vi "aft_ANC_Analyze Residual Siganl.vi"(10 "restart averaging":bool, 11 "signal":fxp<+/-,24,4>[](array[numeric]) format="%.22g") -> (2 "residual noise":dbl[](array[numeric]), 3 "power spectrum":cluster{"f0":dbl, "df":dbl, "magnitude":dbl[]})   [LabVIEW 2019]
uses:
  <vilib>/Analysis/baseanly.llb/IIR Cascade Filter (DBL).vi
  <vilib>/measure/maspectr.llb/FFT Power Spectrum for 1 Chan.vi
  <vilib>/measure/NI_MAPro.lvlib
  <vilib>/Analysis/NI_AALBase.lvlib
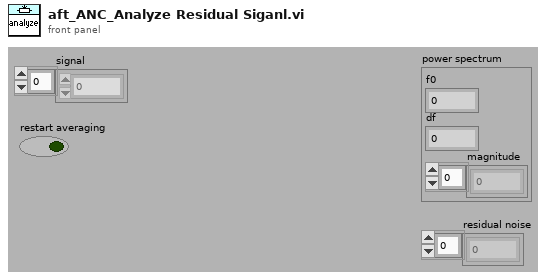
[diagram p1: front panel]
types:
  T1 = enum32{"Lowpass", "Highpass", "Bandpass", "Bandstop"}
  T2 = cluster{"filter structure":enum32{"IIR 2nd Order", "IIR 4th Order"}, "Reverse Coefficients":dbl[], "Forward Coefficients":dbl[]}
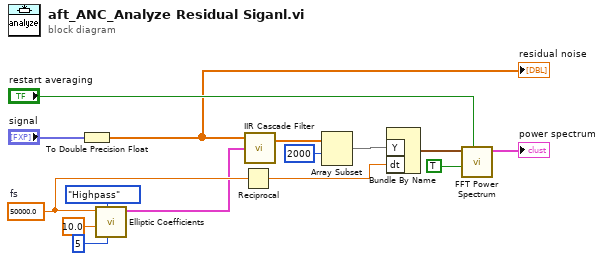
[diagram p0: block diagram]
diagram:
  w3 = 50000.0  # fs
  n1 = To Double Precision Float(number="signal") -> (double precision float=w1:dbl[])
  "residual noise" <- w1
  n2 = call <vilib>:"Elliptic Coefficients.vi"("order"=5, "filter type"=T1."Highpass", "low cutoff freq: fl"=10.0, "sampling freq: fs"=w3) -> ("IIR Filter Cluster"=w2:T2)  [unwired: 6 in, 1 out]
  n3 = Reciprocal(x=w3) -> (1/x=w9:dbl)
  n4 = call-poly <vilib>:"IIR Cascade Filter.vi"("IIR Filter Cluster"=w2, "X"=w1) -> ("Filtered X"=w12:dbl[])  [unwired: 1 in, 1 out]
  n5 = Array Subset(array=w12, index=2000) -> (w14:dbl[])  [unwired: 1 in]
  n6 = Bundle By Name("Y"=w14, "dt"=w9) -> (w7:waveform(dbl))  [unwired: 1 out]
  n7 = call-poly <vilib>:"FFT Power Spectrum.vi"("restart averaging (F)"="restart averaging", "dB On (F)"=TRUE, "time signal"=w7) -> ("power spectrum"=→"power spectrum":cluster{"f0":dbl, "df":dbl, "magnitude":dbl[]})  [unwired: 5 in, 3 out]
